vi "Proceed.vi"(7 "component is ready (Y)":bool=TRUE, 8 "error in (no error)":errorcluster, 10 "ProceedMessage":refnum<class "ProceedMessage.lvclass">, 11 "Autofocus in":refnum<class "Autofocus.lvclass">) -> (0 "error out":errorcluster, 2 "all observers are ready?":bool, 3 "Autofocus out":refnum<class "Autofocus.lvclass">)   [LabVIEW 2012, in "Autofocus.lvclass"]
doc: "The Proceed method is used to check if your component is ready. Also it checks if the observers are ready. When the observers and the component are ready, it sends the proceed to its observee. If it's the highest observee, it distributes a stop command."
uses:
  Autofocus.lvclass
  <vilib>/Distrio/Murmex/ProceedMessage/ProceedMessage.lvclass
  Autofocus.lvclass/Autofocus.ctl
  current activity.ctl
  <vilib>/Distrio/Murmex/StopMessage/StopMessage.lvclass
  <vilib>/Distrio/Murmex/GenericMessage/GenericMessage.lvclass
  <vilib>/Distrio/Murmex/Murmex/Murmex.lvclass
  <vilib>/Distrio/Murmex/Message/Add or replace parameter.vi
panel:
  # "This method is called when the PROCEED\ntrigger is sent. \n\nOverride this method when your component needs to\nrespond to this trigger. \n\nCall parent for proper implementation"
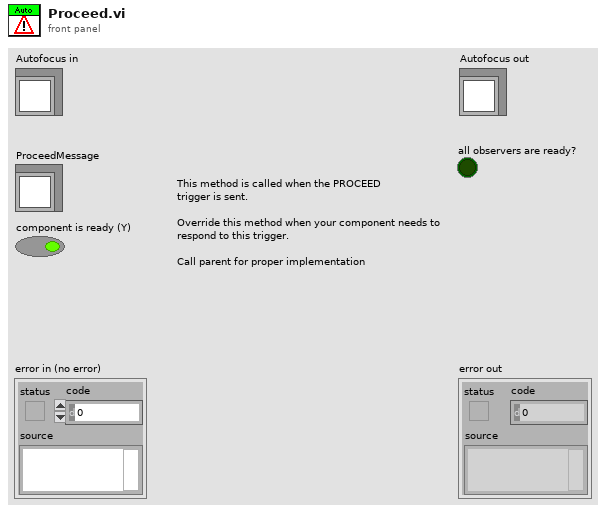
[diagram p1: front panel]
types:
  T1 = typedef "Autofocus.lvclass/current activity.ctl" = enum16{"Image acquisition", "Stack", "Checkpoint", "Idle"}
  T2 = typedef "Autofocus.lvclass/Search algorithm.ctl" = enum16{"Hill Climbing", "HC+GS"}
  T3 = typedef "Autofocus.lvclass/image acquisition mode.ctl" = enum16{"Focus Stack", "Single Frame"}
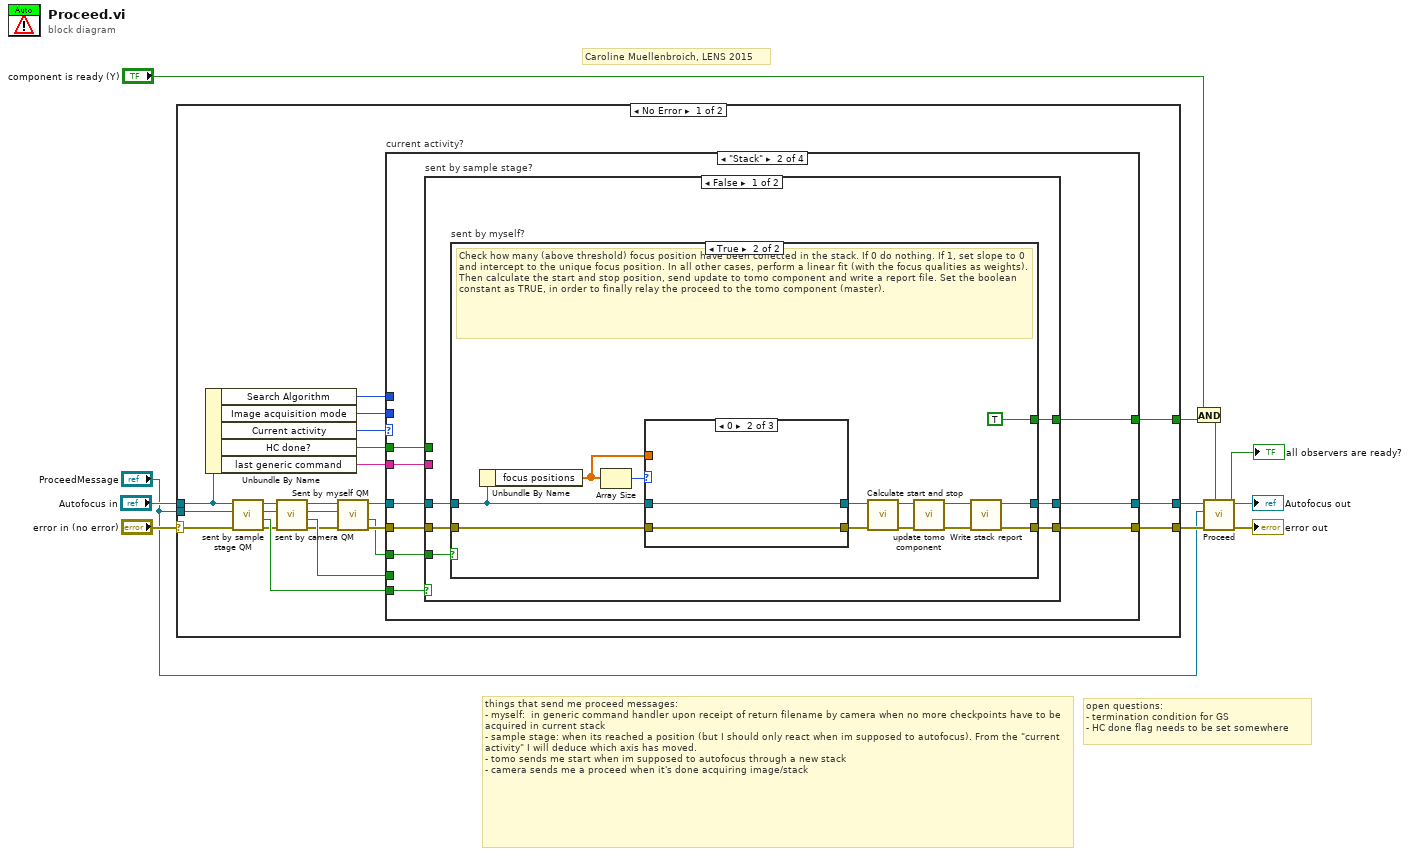
[diagram p0: block diagram]
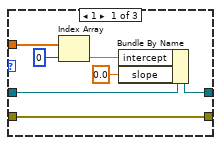
[diagram p4: hidden frame]
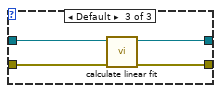
[diagram p5: hidden frame]
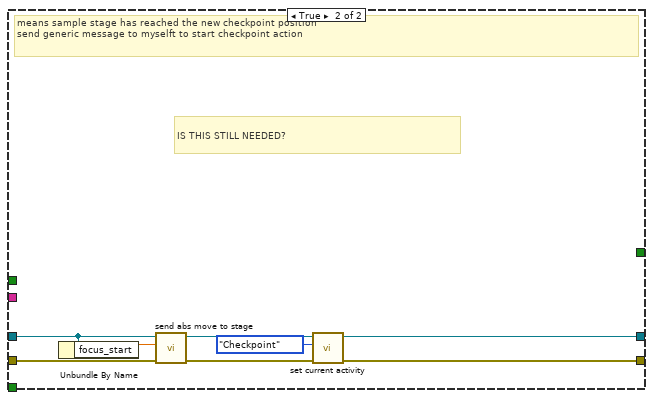
[diagram p6: hidden frame]
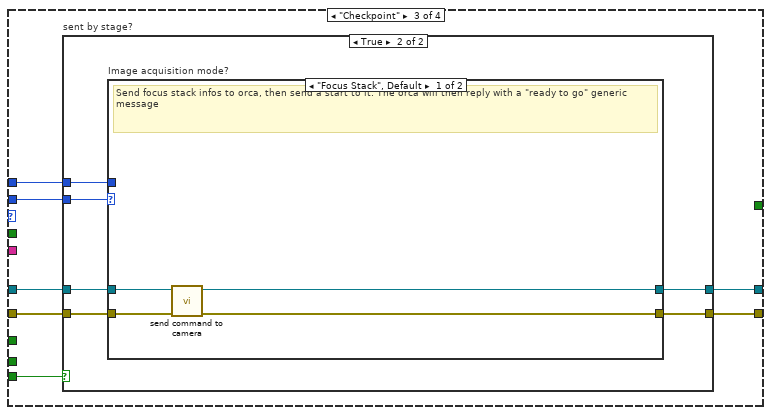
[diagram p7: hidden frame]
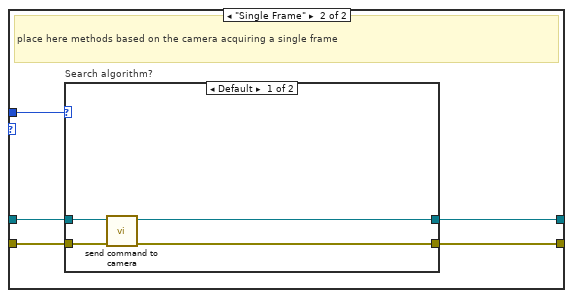
[diagram p9: hidden frame]
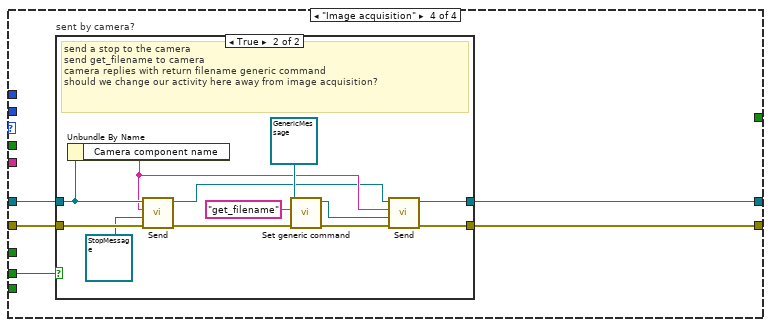
[diagram p11: hidden frame]
diagram:
  # "open questions: \n- termination condition for GS\n- HC done flag needs to be set somewhere"
  # "things that send me proceed messages:\n- myself:  in generic command handler upon receipt of return filename by camera when no more checkpoints have to be acquired in current stack\n- sample stage: when its reached a position (but I should only react when im supposed to autofocus). From the \"current activity\" I will deduce which axis has moved.\n- tomo sends me start when im supposed to autofocus through a new stack\n- camera sends me a proceed when it's done acquiring image/stack"
  # "Caroline Muellenbroich, LENS 2015"
  n1 = case shown="No Error" "error in (no error)" {
    selector: "error in (no error)" -> [w29 w137]
    tunnel: [w33 w137] -> w7
    tunnel: "Autofocus in" -> [w28 w136]
    tunnel: [w32 w136] -> w5
    tunnel: "ProceedMessage" -> [w27 _]
    tunnel: [w12 _] -> w1
    frame No Error {
      n2 = Unbundle By Name(w28) -> ("Search Algorithm"=w22:T2, "Image acquisition mode"=w23:T3, "Current activity"=w24:T1, "HC done?"=w30:bool, "last generic command"=w31:string)
      n3 = call-dynamic "sent by sample stage QM.vi"("error in (no error)"=w29, "ProceedMessage"=w27, "Autofocus in"=w28) -> ("error out"=w25:errorcluster, "sent by sample stage?"=w26:bool, "ProceedMessage 2"=w20:refnum<class "ProceedMessage.lvclass">, "Autofocus out"=w21:refnum<class "Autofocus.lvclass">)  [unwired: 5 in]
      n4 = call-dynamic "sent by camera QM.vi"("error in (no error)"=w25, "ProceedMessage"=w20, "Autofocus in"=w21) -> ("error out"=w18:errorcluster, "sent by camera?"=w19:bool, "ProceedMessage 2"=w14:refnum<class "ProceedMessage.lvclass">, "Autofocus out"=w16:refnum<class "Autofocus.lvclass">)  [unwired: 5 in]
      n5 = call-dynamic "Sent by myself QM.vi"("error in (no error)"=w18, "ProceedMessage"=w14, "Autofocus in"=w16) -> ("error out"=w17:errorcluster, "sent by myself?"=w13:bool, "Autofocus out"=w15:refnum<class "Autofocus.lvclass">)  [unwired: 5 in, 1 out]
      n6 = case "current activity?" shown="\"Stack\"" w24 {
        tunnel: [w34 w44 w87 w120] -> w33
        tunnel: [w35 w43 w88 w118] -> w32
        tunnel: w31 -> [_ w42 _ _]
        tunnel: w30 -> [_ w41 _ _]
        tunnel: w26 -> [_ w40 w93 _]
        tunnel: w15 -> [w35 w39 w89 w117]
        tunnel: w17 -> [w34 w38 w90 w119]
        tunnel: w23 -> [_ _ w92 _]
        tunnel: w22 -> [_ _ w91 _]
        tunnel: w19 -> [_ _ _ w121]
        tunnel: w13 -> [_ w37 _ _]
        tunnel: [_ w36 _ _] -> w12
        frame "Idle", Default {
        }
        frame "Stack" {
          n7 = case "sent by sample stage?" shown="False" w40 {
            tunnel: [w45 w86] -> w44
            tunnel: [w46 w85] -> w43
            tunnel: w42 -> [_ _]
            tunnel: w41 -> [_ _]
            tunnel: w38 -> [w48 w82]
            tunnel: w39 -> [w49 w80]
            tunnel: w37 -> [w50 _]
            tunnel: [w47 _] -> w36
            frame False {
              n8 = case "sent by myself?" shown="True" w50 {
                tunnel: w49 -> [w52 w64]
                tunnel: w48 -> [w51 w65]
                tunnel: [_ TRUE] -> w47
                tunnel: [w52 w53] -> w46
                tunnel: [w51 w55] -> w45
                frame False {
                }
                frame True {
                  # "Check how many (above threshold) focus position have been collected in the stack. If 0 do nothing. If 1, set slope to 0 and intercept to the unique focus position. In all other cases, perform a linear fit (with the focus qualities as weights). Then calculate the start and stop position, send update to tomo component and write a report file. Set the boolean constant as TRUE, in order to finally relay the proceed to the tomo component (master)."
                  n9 = Unbundle By Name(w64) -> ("focus positions"=w63:dbl[])
                  n10 = Array Size(array=w63) -> (size(s)=w62:i32)
                  n11 = case shown="0" w62 {
                    tunnel: w65 -> [w66 w73 w78]
                    tunnel: w64 -> [w70 w74 w77]
                    tunnel: [w67 w74 w76] -> w60
                    tunnel: [w66 w73 w75] -> w61
                    tunnel: w63 -> [w72 _ _]
                    frame 1 {
                      n12 = Index Array(array=w72, index=0 ("y")) -> (element=w69:dbl)
                      n13 = Bundle By Name(cluster=w70, "intercept"=w69, "slope"=0.0 ("Runtime cluster.Stack.slope")) -> (w67:refnum<class "Autofocus.lvclass">)
                    }
                    frame 0 {
                    }
                    frame Default {
                      n14 = call-dynamic "calculate linear fit.vi"("error in (no error)"=w78, "Autofocus in"=w77) -> ("error out"=w75:errorcluster, "Autofocus out"=w76:refnum<class "Autofocus.lvclass">)  [unwired: 8 in]
                    }
                  }
                  n15 = call-dynamic "Calculate start and stop.vi"("error in (no error)"=w61, "Autofocus in"=w60) -> ("error out"=w59:errorcluster, "Autofocus out"=w58:refnum<class "Autofocus.lvclass">)  [unwired: 8 in]
                  n16 = call-dynamic "update tomo component.vi"("error in (no error)"=w59, "Autofocus in"=w58) -> ("error out"=w56:errorcluster, "Autofocus out"=w54:refnum<class "Autofocus.lvclass">)  [unwired: 8 in]
                  n17 = call-dynamic "Write stack report.vi"("error in (no error)"=w56, "Autofocus in"=w54) -> ("error out"=w55:errorcluster, "Autofocus out"=w53:refnum<class "Autofocus.lvclass">)  [unwired: 8 in]
                }
              }
            }
            frame True {
              # "IS THIS STILL NEEDED?"
              # "means sample stage has reached the new checkpoint position\nsend generic message to myselft to start checkpoint action"
              n18 = Unbundle By Name(w80) -> ("focus_start"=w79:dbl[unit])
              n19 = call-dynamic "send abs move to stage.vi"("error in (no error)"=w82, "absolute z position"=w79, "Autofocus in"=w80) -> ("error out"=w81:errorcluster, "Autofocus out"=w83:refnum<class "Autofocus.lvclass">)  [unwired: 7 in]
              n20 = call-dynamic "set current activity.vi"("error in (no error)"=w81, "Current activity"=current_activity."Checkpoint", "Autofocus in"=w83) -> ("error out"=w86:errorcluster, "Autofocus out"=w85:refnum<class "Autofocus.lvclass">)  [unwired: 7 in]
            }
          }
        }
        frame "Checkpoint" {
          n21 = case "sent by stage?" shown="True" w93 {
            tunnel: w92 -> [_ w101]
            tunnel: w91 -> [_ w100]
            tunnel: w90 -> [w94 w99]
            tunnel: w89 -> [w95 w98]
            tunnel: [w95 w97] -> w88
            tunnel: [w94 w96] -> w87
            frame False {
            }
            frame True {
              n22 = case "Image acquisition mode?" shown="\"Focus Stack\", Default" w101 {
                tunnel: w100 -> [_ w110]
                tunnel: w99 -> [w105 w109]
                tunnel: w98 -> [w104 w107]
                tunnel: [w103 w106] -> w97
                tunnel: [w102 w108] -> w96
                frame "Focus Stack", Default {
                  # "Send focus stack infos to orca, then send a start to it. The orca will then reply with a \"ready to go\" generic message"
                  n23 = call-dynamic "send command to camera.vi"("error in (no error)"=w105, "Autofocus in"=w104) -> ("error out"=w102:errorcluster, "Autofocus out"=w103:refnum<class "Autofocus.lvclass">)  [unwired: 8 in]
                }
                frame "Single Frame" {
                  # "place here methods based on the camera acquiring a single frame"
                  n24 = case "Search algorithm?" shown="Default" w110 {
                    tunnel: w109 -> [w114 w116]
                    tunnel: [w113 w116] -> w108
                    tunnel: w107 -> [w112 w115]
                    tunnel: [w111 w115] -> w106
                    frame Default {
                      n25 = call-dynamic "send command to camera.vi"("error in (no error)"=w114, "Autofocus in"=w112) -> ("error out"=w113:errorcluster, "Autofocus out"=w111:refnum<class "Autofocus.lvclass">)  [unwired: 8 in]
                    }
                    frame "Hill Climbing" {
                    }
                  }
                }
              }
            }
          }
        }
        frame "Image acquisition" {
          n26 = case "sent by camera?" shown="True" w121 {
            tunnel: [w123 w124] -> w120
            tunnel: w119 -> [w123 w135]
            tunnel: [w122 w125] -> w118
            tunnel: w117 -> [w122 w134]
            frame False {
              # "Just ignore it. It probably is sent from the stage in case of stack acquisition"
            }
            frame True {
              # "send a stop to the camera\nsend get_filename to camera\ncamera replies with return filename generic command\nshould we change our activity here away from image acquisition?"
              n27 = Unbundle By Name(w134) -> ("Camera component name"=w127:string)
              n28 = call <vilib>:"Send.vi"("error in (no error)"=w135, "Message"=refnum<class "StopMessage.lvclass"> refnum ("Message in"), "recipient"=w127, "Murmex in"=w134) -> ("error out"=w132:errorcluster, "Murmex out"=w126:refnum<class "Autofocus.lvclass">)  [unwired: 6 in]
              n29 = call <vilib>:"Set generic command.vi"("error in (no error)"=w132, "generic command"="get_filename", "GenericMessage in"=refnum<class "GenericMessage.lvclass"> refnum ("Distrio Murmex 1.5:GenericMessage")) -> ("error out"=w131:errorcluster, "GenericMessage out"=w128:refnum<class "GenericMessage.lvclass">)  [unwired: 7 in]
              n30 = call <vilib>:"Send.vi"("error in (no error)"=w131, "Message"=w128, "recipient"=w127, "Murmex in"=w126) -> ("error out"=w124:errorcluster, "Murmex out"=w125:refnum<class "Autofocus.lvclass">)  [unwired: 6 in]
            }
          }
        }
      }
    }
    frame Error {
    }
  }
  n31 = And(x="component is ready (Y)", y=w1) -> (x .and. y?=w2:bool)
  n32 = call-parent "Proceed.vi"("component is ready (Y)"=w2, "error in (no error)"=w7, "ProceedMessage"="ProceedMessage", "Murmex in"=w5) -> ("error out"=→"error out":errorcluster, "all observers are ready?"=→"all observers are ready?":bool, "Murmex out"=→"Autofocus out":refnum<class "Autofocus.lvclass">)  [unwired: 5 in]
